vi "Configure Session.vi"(8 "error in":errorcluster, 11 "Plugin in":refnum<class "Historical Table.lvclass">) -> (0 "error out":errorcluster, 3 "Plugin out":refnum<class "Historical Table.lvclass">)   [LabVIEW 2024, in "Historical Table.lvlib" / "Historical Table.lvclass"]
uses:
  Historical Table.lvclass
  C:/Program Files/National Instruments/LabVIEW 2024/vi.lib/FlexLogger/SDK/PluginSDK.lvlibp/PEFClasses/SDK/Plugin/Plugin.lvclass
  Historical Table.lvclass/Historical Table.ctl
  Global Strings.vi
  <vilib>/FlexLogger/SDK/PluginSDK.lvlibp/PEFClasses/SDK/Plugin/ParameterAccess/Read I32.vi
  <vilib>/FlexLogger/SDK/PluginSDK.lvlibp/PEFClasses/SDK/Plugin/ParameterAccess/Write I32.vi
  <vilib>/FlexLogger/SDK/PluginSDK.lvlibp/PEFClasses/SDK/Plugin/Get Valid Consumer Channels.vi
  <vilib>/FlexLogger/SDK/PluginSDK.lvlibp/PEFClasses/SDK/Consumer Channel/Consumer Channel.lvclass
  <vilib>/FlexLogger/SDK/PluginSDK.lvlibp/PEFClasses/SDK/Plugin/Plugin.lvclass
  C:/Program Files/National Instruments/LabVIEW 2024/vi.lib/FlexLogger/SDK/PluginSDK.lvlibp/PEFClasses/SDK/Processing Element/Processing Element.lvclass
  C:/Users/bbuchana/Documents/LabVIEW Projects/FlexLogger IO Plug-ins/Historical Table/Historical Table.lvclass
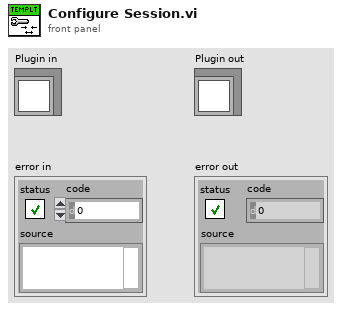
[diagram p1: front panel]
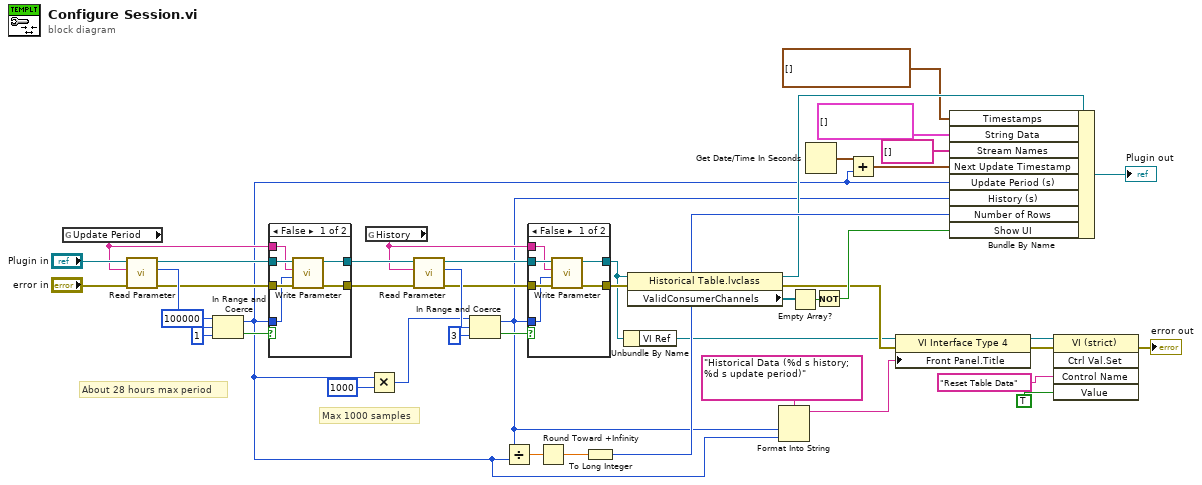
[diagram p0: block diagram]
diagram:
  # "Max 1000 samples"
  # "About 28 hours max period"
  n1 = global read "Global Strings.vi" "Update Period"() -> (w35:string)
  n2 = call-poly <vilib>:"Read Parameter.vi"("error in (no error)"="error in", "Name"=w35, "Plugin in"="Plugin in") -> ("error out"=w36:errorcluster, "Value"=w39:i32, "Plugin out"=w37:refnum<class "Historical Table.lvclass">)  [unwired: 5 in, 1 out]
  n3 = In Range and Coerce(upper limit=100000, x=w39, lower limit=1) -> (coerced(x)=w11:i32, In Range?=w38:bool)
  n4 = case shown="False" w38 {
    tunnel: w37 -> [w51 w53]
    tunnel: [w47 w53] -> w34
    tunnel: w36 -> [w50 w52]
    tunnel: w11 -> [w48 _]
    tunnel: [w46 w52] -> w33
    tunnel: w35 -> [w49 _]
    frame False {
      n5 = call-poly <vilib>:"Write Parameter.vi"("error in (no error)"=w50, "Value"=w48, "Name"=w49, "Plugin in"=w51) -> ("error out"=w46:errorcluster, "Plugin out"=w47:refnum<class "Historical Table.lvclass">)  [unwired: 6 in]
    }
    frame True {
    }
  }
  n6 = global read "Global Strings.vi" "History"() -> (w28:string)
  n7 = Multiply(x=w11, y=1000) -> (x*y=w31:i32)
  n8 = call-poly <vilib>:"Read Parameter.vi"("error in (no error)"=w33, "Name"=w28, "Plugin in"=w34) -> ("error out"=w27:errorcluster, "Value"=w45:i32, "Plugin out"=w29:refnum<class "Historical Table.lvclass">)  [unwired: 5 in, 1 out]
  n9 = In Range and Coerce(upper limit=w31, x=w45, lower limit=3) -> (coerced(x)=w13:i32, In Range?=w30:bool)
  n10 = Divide(x=w13, y=w11) -> (x/y=w26:dbl)
  n11 = case shown="False" w30 {
    tunnel: w29 -> [w59 w61]
    tunnel: [w55 w61] -> w15
    tunnel: w27 -> [w58 w60]
    tunnel: w13 -> [w56 _]
    tunnel: [w54 w60] -> w23
    tunnel: w28 -> [w57 _]
    frame False {
      n12 = call-poly <vilib>:"Write Parameter.vi"("error in (no error)"=w58, "Value"=w56, "Name"=w57, "Plugin in"=w59) -> ("error out"=w54:errorcluster, "Plugin out"=w55:refnum<class "Historical Table.lvclass">)  [unwired: 6 in]
    }
    frame True {
    }
  }
  n13 = Round Toward +Infinity(x=w26) -> (ceil(x): smallest int >= x=w25:dbl)
  n14 = To Long Integer(number=w25) -> (32bit integer=w24:i32)
  n15 = Unbundle By Name(w15) -> ("VI Ref"=w6:refnum<vi>)
  n16 = property class="Historical Table.lvclass"(reference=w15, error in=w23) -> (reference out=w21:refnum<class "Historical Table.lvclass">, error out=w7:errorcluster, "ValidConsumerChannels"=w9:refnum<class "Consumer Channel.lvclass">[])
  n17 = Format Into String(format string="Historical Data (%d s history; %d s update period)", w13, w11) -> (resulting string=w12:string)  [unwired: 2 in, 1 out]
  n18 = Empty Array?(array=w9) -> (empty?=w22:bool)
  n19 = Get Date/Time In Seconds() -> (seconds since 1Jan1904=w17:timestamp)
  n20 = Not(x=w22) -> (.not. x?=w10:bool)
  n21 = Add(x=w17, y=w11) -> (x+y=w16:timestamp)
  n22 = property class="VI Interface Type 4"(reference=w6, error in=w7, "Front Panel.Title"=w12) -> (reference out=w5:refnum<vi>, error out=w4:errorcluster)
  n23 = Bundle By Name(cluster=w21, "Timestamps"=timestamp[] [], "String Data"=cluster{"Data":string[]}[] [], "Stream Names"=string[] [], "Next Update Timestamp"=w16, "Update Period (s)"=w11, "History (s)"=w13, "Number of Rows"=w24, "Show UI"=w10) -> (→"Plugin out":refnum<class "Historical Table.lvclass">)
  n24 = invoke class="VI (strict)" method="Ctrl Val.Set"(reference=w5, error in=w4, "Control Name"="Reset Table Data", "Value"=TRUE ("Reset Table Data")) -> (error out=→"error out":errorcluster)  [unwired: 1 in, 4 out]
